vi "DetermineDesiredRegime.vi"(9 "Altered regime boundaries":T1=[0, 70, 140, 220, 190, 290], 10 "Desired Heading (deg)":dbl, 11 "Trusted Absolute Wind Data (deg)":dbl) -> (3 "Sailing Regime":T2)   [LabVIEW 2013]
doc: "This VI looks at the desired robot heading and compares it against the wind, then determines which boat regime we want to be in, ignoring whether or not we want to transition. It ignores the transistions because another section of the code checks whether our desired regime and actual regime differand require a transition.\n\nEric Schneider, Feb. 2014"
uses:
  Data/TypeDefs/Sailing Regimes.ctl
  Data/TypeDefs/Regime Boundaries.ctl
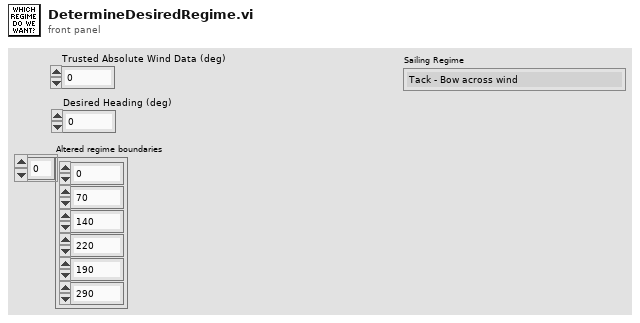
[diagram p1: front panel]
types:
  T1 = typedef "Regime Boundaries.ctl" = i32[]
  T2 = typedef "Sailing Regimes.ctl" = enum16{"Tack - Bow across wind", "Upwind - Port Tack", "Turn between Upwind/Reach - Port Tack", "Reach - Port Tack", "Turn between Reach/Run - Port Tack", "Run - Port Tack", "Jibe - Stern across wind", "Run - Starboard Tack", "Turn between Reach/Run - Starboard Tack", "Reach - Starboard Tack", "Turn between Upwind/Reach - Starboard Tack", "Upwind - Starboard Tack"}
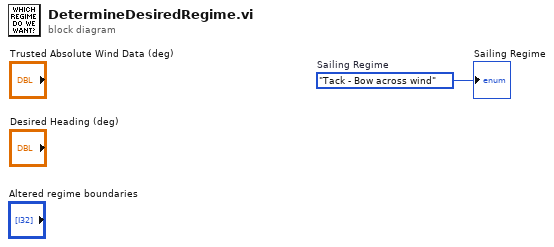
[diagram p0: block diagram]
diagram:
  w1 = Sailing_Regimes."Tack - Bow across wind"  # Sailing Regime
  "Sailing Regime" <- w1
